vi "Get Type.vi"(11 "Path in":refnum<class "Path.lvclass">) -> (3 "Type":string)   [LabVIEW 2017, in "Path.lvclass"]
uses:
  <vilib>/gpm_packages/@cs/data-type-serializer/source/Path/Path.lvclass
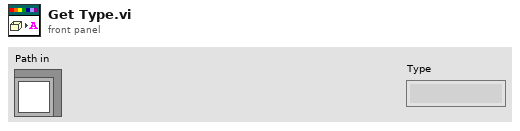
[diagram p1: front panel]
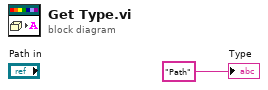
[diagram p0: block diagram]
diagram:
  "Type" <- "Path" ("Type")
